vi "midterm2.vi"() -> ()   [LabVIEW 2009]
panel:
  in  "?":bool
  in  "Enter Password":string
  out "Arm Countdown":i32
  out "Front door indicator":bool[](array[boolean])
  out "Alarm Countdown":i32
  out "Alarm":bool
  out "On indicates open":bool[](array[boolean])
  in  "Disarm":bool
  out "Armed":bool
  in  "?":bool
  # "Burglar Alarm System"
  # "Window 1"
  # "Window 2"
  # "Back door"
  # "Front door"
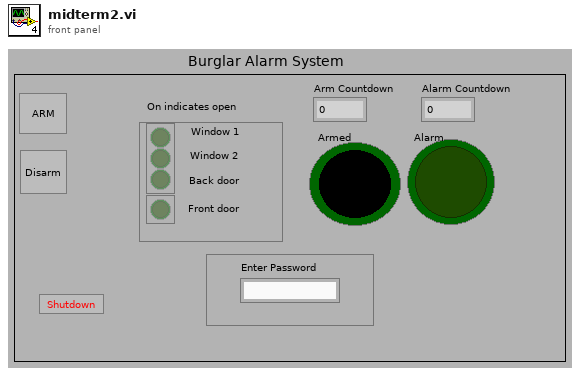
[diagram p1: front panel]
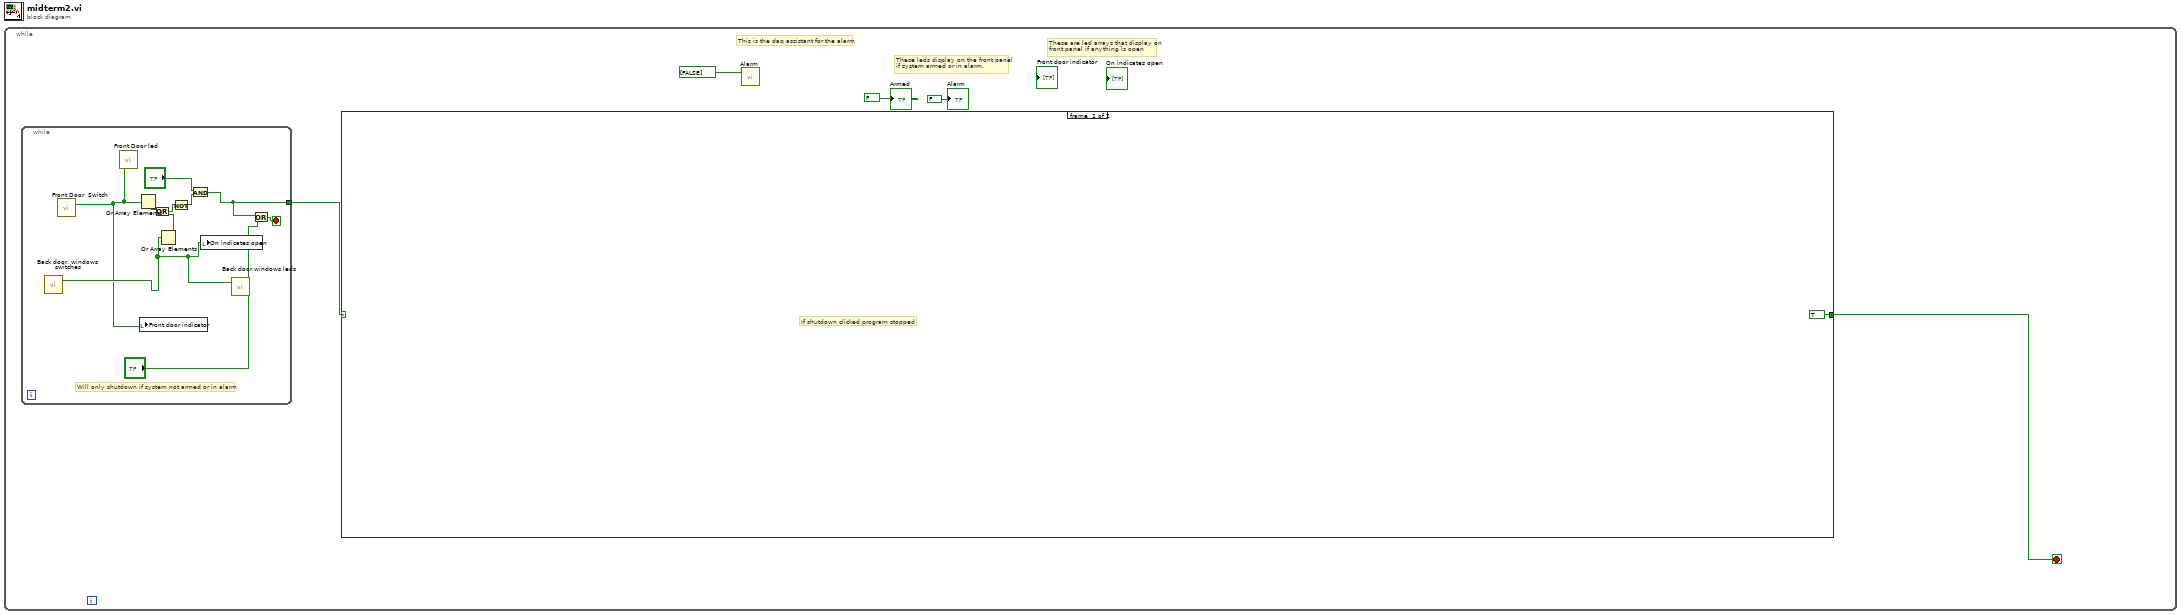
[diagram p0: block diagram]
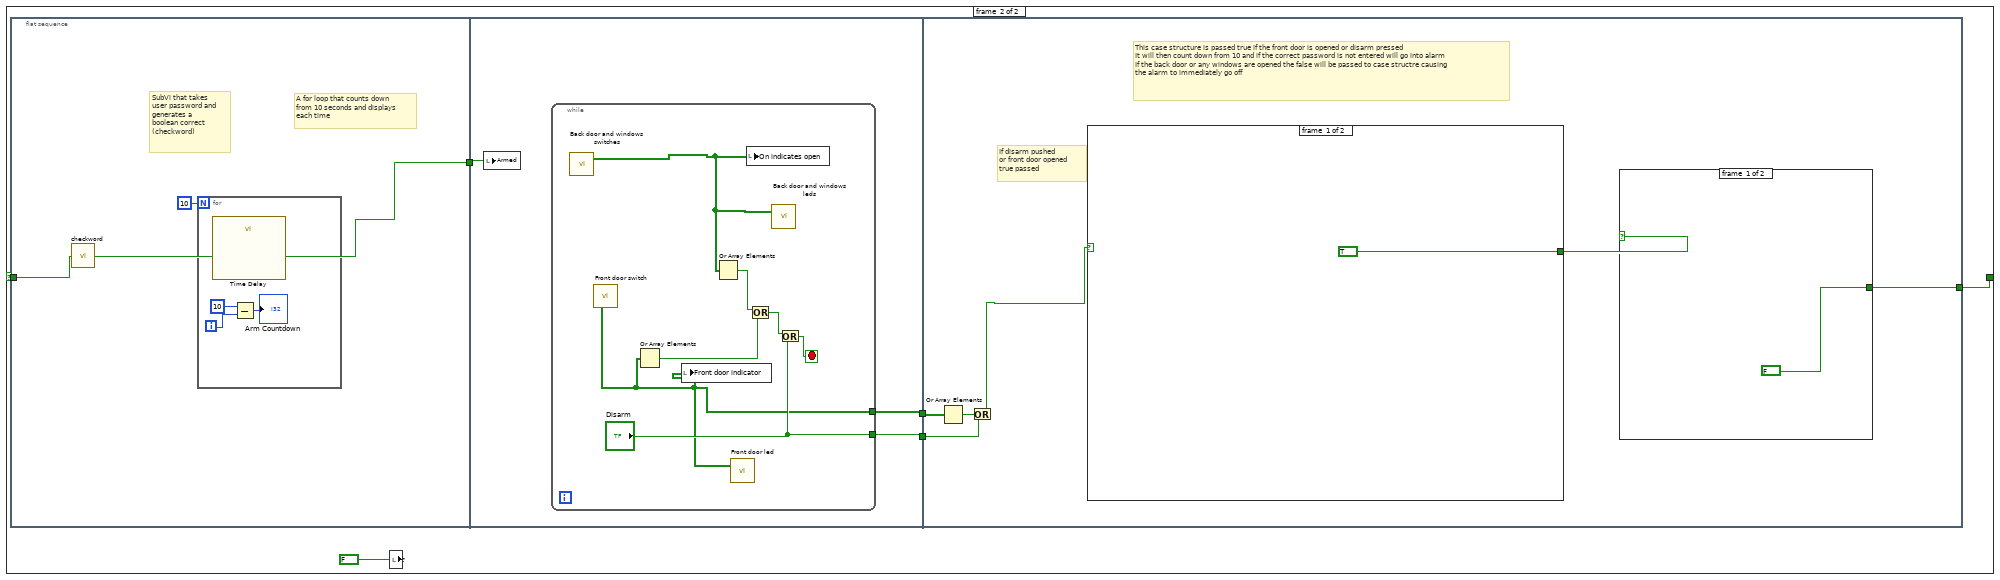
[diagram p2: hidden frame]
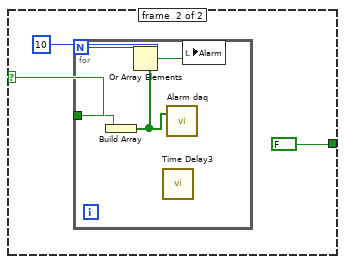
[diagram p3: hidden frame]
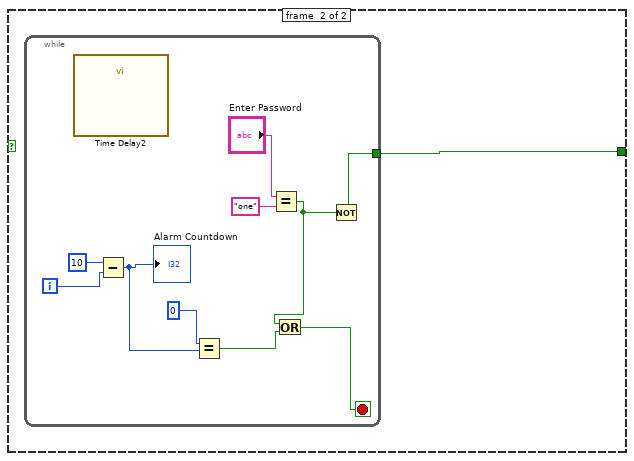
[diagram p4: hidden frame]
diagram:
  n1 = while {
    stop <- w1 stop-if-true
    # "This is the daq assistant for the alarm"
    # "These are led arrays that display on\nfront panel if anything is open"
    # "These leds display on the front panel\nif system armed or in alarm."
    n2 = while {
      tunnel: [w8] -> w2
      stop <- w7 stop-if-true
      # "Will only shutdown if system not armed or in alarm"
      n3 = call "Back door, windows switches"() -> ("data"=w10:bool[])  [unwired: 17 in, 2 out]
      n4 = call "Front Door  Switch"() -> ("data"=w9:bool[])  [unwired: 17 in, 2 out]
      n5 = call "Front Door led"("data"=w9) -> ()  [unwired: 17 in, 2 out]
      n6 = Or Array Elements(Boolean array=w9) -> (logical OR=w13:bool)
      n7 = local write "Front door indicator"(w9) -> ()
      n8 = Or Array Elements(Boolean array=w10) -> (logical OR=w12:bool)
      n9 = Or(x=w13, y=w12) -> (x .or. y?=w11:bool)
      n10 = Not(x=w11) -> (.not. x?=w14:bool)
      n11 = And(x="?", y=w14) -> (x .and. y?=w8:bool)
      n12 = local write "On indicates open"(w10) -> ()
      n13 = call "Back door,windows leds"("data"=w10) -> ()  [unwired: 17 in, 2 out]
      n14 = Or(x=w8, y="?") -> (x .or. y?=w7:bool)
    }
    n15 = case shown="True" w2 {
      selector: w2 -> [_ w18]
      tunnel: [TRUE ("Stop Program") w17] -> w1
      frame #0 {
        # "If shutdown clicked program stopped"
      }
      frame #1 {
        n16 = flat-sequence {
          tunnel: [w25] -> w22
          tunnel: w18 -> [w23]
          tunnel: [w31] -> w21
          tunnel: [w30] -> w20
          tunnel: w22 -> [w29]
          tunnel: w21 -> [w44]
          tunnel: w20 -> [w42]
          tunnel: [w39] -> w17
          frame #0 {
            # "SubVi that takes user password and \ngenerates a boolean correct\n(checkword)"
            # "A for loop that counts down\nfrom 10 seconds and displays\neach time"
            n17 = call "checkword.vi"("Enable"=w23) -> ("Boolean"=w25:bool)
            n18 = for {
              N: 10 -> [_]
              i -> [w28]
              n19 = call "Time Delay"() -> ()  [unwired: 11 in, 1 out]
              n20 = Subtract(x=10, y=w28) -> (x-y=→"Arm Countdown":i32)
            }
          }
          frame #1 {
            n21 = local write "Armed"(w29) -> ()
            n22 = while {
              tunnel: [w32] -> w31
              tunnel: ["Disarm"] -> w30
              stop <- w35 stop-if-true
              n23 = call "Back door and windows switches"() -> ("data"=w33:bool[])  [unwired: 17 in, 2 out]
              n24 = call "Front door switch"() -> ("data"=w32:bool[])  [unwired: 17 in, 2 out]
              n25 = Or Array Elements(Boolean array=w32) -> (logical OR=w37:bool)
              n26 = local write "Front door indicator"(w32) -> ()
              n27 = Or Array Elements(Boolean array=w33) -> (logical OR=w38:bool)
              n28 = call "Front door led"("data"=w32) -> ()  [unwired: 17 in, 2 out]
              n29 = local write "On indicates open"(w33) -> ()
              n30 = Or(x=w38, y=w37) -> (x .or. y?=w36:bool)
              n31 = call "Back door and windows leds"("data"=w33) -> ()  [unwired: 17 in, 2 out]
              n32 = Or(x=w36, y="Disarm") -> (x .or. y?=w35:bool)
            }
          }
          frame #2 {
            # "If disarm pushed\nor front door opened\ntrue passed"
            # "This case structure is passed true if the front door is opened or disarm pressed\nIt will then count down from 10 and if the correct password is not entered will go into alarm\nIf the back door or any windows are opened the false will be passed to case structre causing \nthe alarm to immediately go off"
            n33 = Or Array Elements(Boolean array=w44) -> (logical OR=w43:bool)
            n34 = Or(x=w42, y=w43) -> (x .or. y?=w41:bool)
            n35 = case shown="True" w41 {
              tunnel: [TRUE ("Alarm") w53] -> w40
              frame #0 {
              }
              frame #1 {
                n36 = while {
                  tunnel: [w54] -> w53
                  i -> [w63]
                  stop <- w56 stop-if-true
                  n37 = call "Time Delay2"() -> ()  [unwired: 11 in, 1 out]
                  n38 = Subtract(x=10, y=w63) -> (x-y=w61:i32)
                  "Alarm Countdown" <- w61
                  n39 = Equal?(x=0, y=w61) -> (x = y?=w57:bool)
                  n40 = Equal?(x="Enter Password", y="one") -> (x = y?=w55:bool)
                  n41 = Or(x=w55, y=w57) -> (x .or. y?=w56:bool)
                  n42 = Not(x=w55) -> (.not. x?=w54:bool)
                }
              }
            }
            n43 = case shown="True" w40 {
              selector: w40 -> [_ w47]
              tunnel: [FALSE ("Stop Program") FALSE ("Stop Program")] -> w39
              frame #0 {
              }
              frame #1 {
                n44 = for {
                  N: 10 -> [_]
                  tunnel: w47 -> [w50]
                  n45 = Build Array(w50) -> (w49:bool[])
                  n46 = Or Array Elements(Boolean array=w49) -> (logical OR=w51:bool)
                  n47 = call "Time Delay3"() -> ()  [unwired: 11 in, 1 out]
                  n48 = call "Alarm daq"("data"=w49) -> ()  [unwired: 17 in, 2 out]
                  n49 = local write "Alarm"(w51) -> ()
                }
              }
            }
          }
        }
        n50 = local write item#9(FALSE ("Stop Pressed")) -> ()
      }
    }
    n51 = call "Alarm"("data"=bool[] [FALSE]) -> ()  [unwired: 17 in, 2 out]
    "Armed" <- FALSE ("Armed")
    "Alarm" <- FALSE ("Alarm")
  }
